vi "calc_vector_length.vi"(1 "vector":cluster{"x":dbl, "y":dbl}) -> (0 "length":dbl)   [LabVIEW 2023]
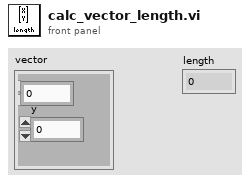
[diagram p1: front panel]
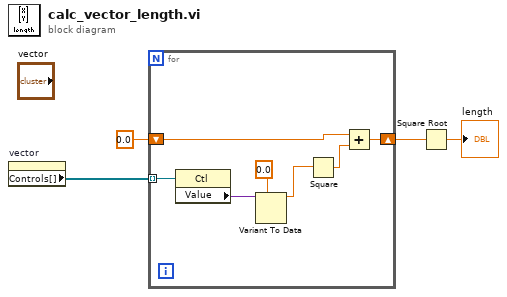
[diagram p0: block diagram]
diagram:
  n1 = property on="vector" class="Clust (strict)"() -> ("Controls[]"=w4:refnum<vi>[])  [unwired: 2 in, 2 out]
  n2 = for {
    tunnel: w4 -> [w11] mode=indexing
    shift-right: [w5] -> w2
    shift-left: 0.0 -> [w6]
    n3 = property class="Ctl"(reference=w11) -> ("Value"=w10:variant)  [unwired: 1 in, 2 out]
    n4 = Variant To Data(type=0.0, Variant=w10) -> (data=w9:dbl)  [unwired: 1 in, 1 out]
    n5 = Square(x=w9) -> (x^2=w7:dbl)
    n6 = Add(x=w6, y=w7) -> (x+y=w5:dbl)
  }
  n7 = Square Root(x=w2) -> (sqrt(x)=→"length":dbl)
